vi "Set FTDI LatencyTimer.vi"() -> ()   [LabVIEW 2013]
uses:
  <vilib>/registry/registry.llb/Registry RtKey.ctl
  <vilib>/registry/registry.llb/Registry SAM.ctl
  <vilib>/registry/registry.llb/Read Registry Value Simple U32.vi
  <vilib>/registry/registry.llb/Read Registry Value Simple STR.vi
  <vilib>/registry/registry.llb/Write Registry Value Simple U32.vi
  <vilib>/regexp/Match Regular Expression.xnode
panel:
  out "New LatencyTimer List":u32[](array[numeric])
  out "Device Registry List":string[](array[string])
  out "# of Connected FTDI Devices":u32
  in  "LatencyTimer":i32=1
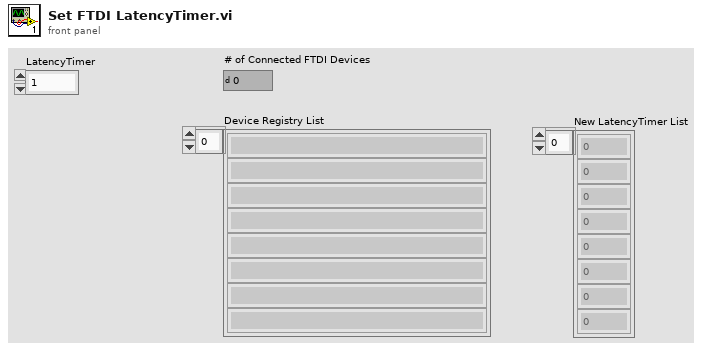
[diagram p1: front panel]
types:
  T1 = typedef "Registry SAM.ctl" = enum32{"KEY_QUERY_VALUE", "KEY_SET_VALUE", "KEY_CREATE_SUB_KEY", "KEY_ENUMERATE_SUB_KEYS", "KEY_NOTIFY", "KEY_CREATE_LINK", "KEY_READ", "KEY_WRITE", "KEY_ALL_ACCESS", "KEY_READ | KEY_WRITE"}
  T2 = typedef "Registry RtKey.ctl" = enum32{"HKEY_CLASSES_ROOT", "HKEY_CURRENT_USER", "HKEY_LOCAL_MACHINE", "HKEY_USERS", "HKEY_PERFORMANCE_DATA", "HKEY_CURRENT_CONFIG", "HKEY_DYN_DATA"}
  T3 = typedef "Registry refnum.ctl" = refnum<k1>
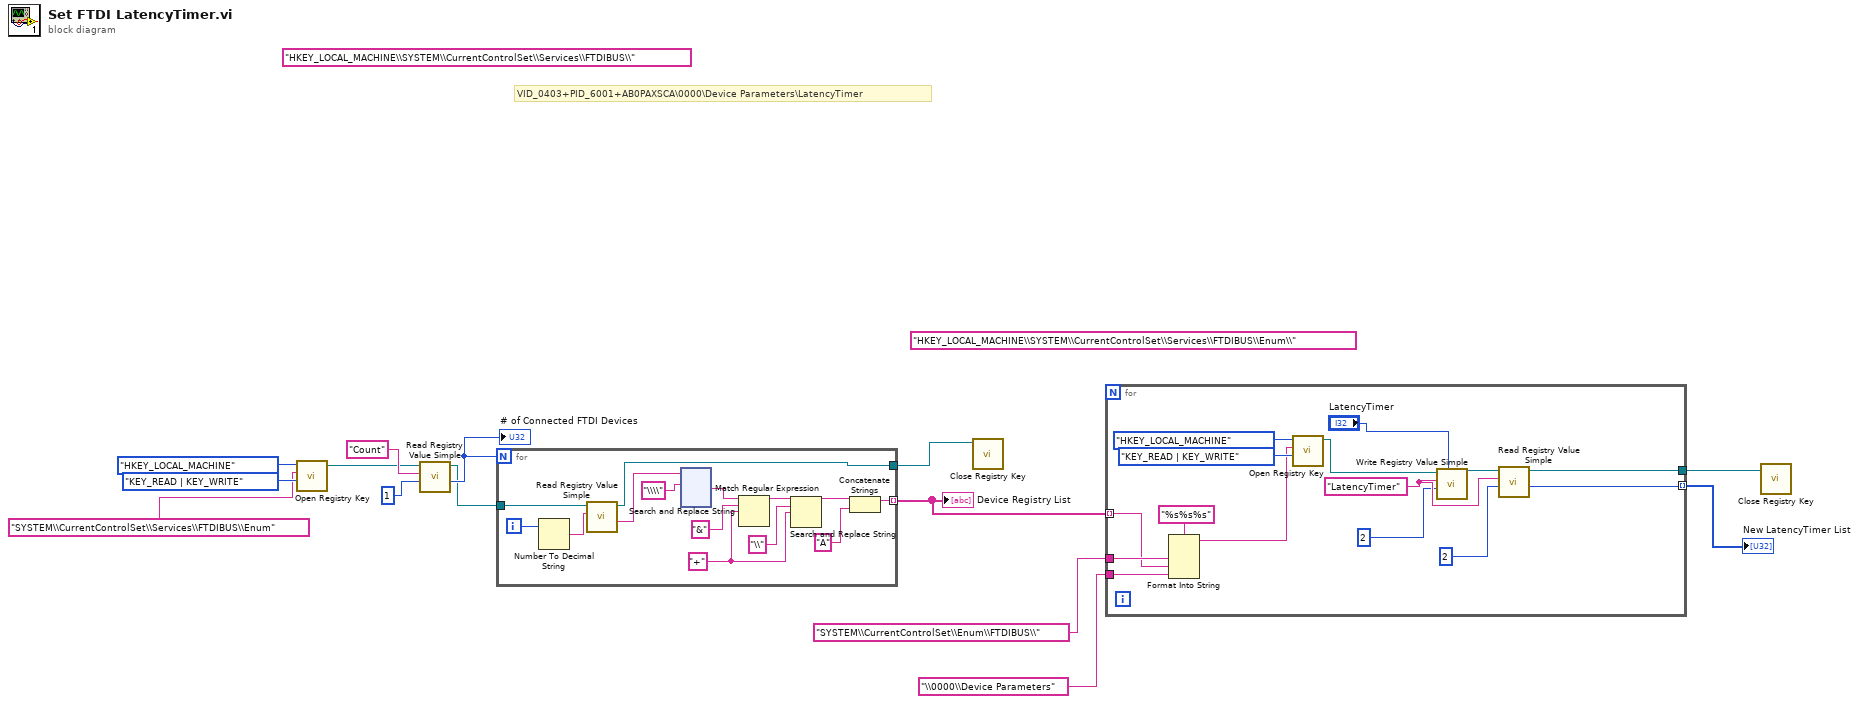
[diagram p0: block diagram]
diagram:
  (unwired) "HKEY_LOCAL_MACHINE\\SYSTEM\\CurrentControlSet\\Services\\FTDIBUS\\Enum\\" ("subkey")
  (unwired) "HKEY_LOCAL_MACHINE\\SYSTEM\\CurrentControlSet\\Services\\FTDIBUS\\" ("subkey")
  # "VID_0403+PID_6001+AB0PAXSCA\\0000\\Device Parameters\\LatencyTimer"
  n1 = call <vilib>:"Open Registry Key.vi"("security access mask (KEY_READ | KEY_WRITE)"=Registry_SAM."KEY_READ | KEY_WRITE", "subkey"="SYSTEM\\CurrentControlSet\\Services\\FTDIBUS\\Enum", "root key (HKEY_LOCAL_MACHINE)"=Registry_RtKey."HKEY_LOCAL_MACHINE") -> ("refnum out"=w10:T3)  [unwired: 7 in, 1 out]
  n2 = call-poly <vilib>:"Read Registry Value Simple.vi"("default data"=1, "value"="Count", "refnum"=w10) -> ("DWORD data"=w8:u32, "refnum out"=w7:T3)  [unwired: 3 in, 2 out]
  "# of Connected FTDI Devices" <- w8
  n3 = for {
    N: w8 -> [_]
    tunnel: w7 -> [w27]
    tunnel: [w15] -> w4 mode=indexing
    tunnel: [w18] -> w1
    i -> [w28]
    w20 = "+" ("search string")
    n4 = Number To Decimal String(number=w28) -> (decimal integer string=w26:string)  [unwired: 1 in]
    n5 = call-poly <vilib>:"Read Registry Value Simple.vi"("value"=w26, "refnum"=w27) -> ("String/Binary data"=w25:string, "refnum out"=w18:T3)  [unwired: 4 in, 2 out]
    n6 = xnode "Match Regular Expression"("input string"=w25, "regular expression"="\\\\") -> ("after match"=w24:string)  [unwired: 4 in, 4 out]
    n7 = Search and Replace String(input string=w24, search string="&" ("replace string (\"\")"), replace string=w20) -> (result string=w23:string)  [unwired: 5 in, 3 out]
    n8 = Search and Replace String(input string=w23, search string="\\", replace string=w20) -> (result string=w17:string)  [unwired: 5 in, 3 out]
    n9 = Concatenate Strings(w17, "A" ("string")) -> (w15:string)
  }
  "Device Registry List" <- w4
  n10 = call <vilib>:"Close Registry Key.vi"("refnum"=w1) -> ()  [unwired: 6 in, 1 out]
  n11 = for {
    tunnel: "SYSTEM\\CurrentControlSet\\Enum\\FTDIBUS\\" -> [w156]
    tunnel: "\\0000\\Device Parameters" -> [w155]
    tunnel: w4 -> [w151] mode=indexing
    tunnel: [w145] -> w3 mode=indexing
    tunnel: [w144] -> w2
    w147 = "LatencyTimer" ("value")
    n12 = Format Into String(format string="%s%s%s", w156, w151, w155) -> (resulting string=w152:string)  [unwired: 2 in, 1 out]
    n13 = call <vilib>:"Open Registry Key.vi"("security access mask (KEY_READ | KEY_WRITE)"=Registry_SAM."KEY_READ | KEY_WRITE", "subkey"=w152, "root key (HKEY_LOCAL_MACHINE)"=Registry_RtKey."HKEY_LOCAL_MACHINE") -> ("refnum out"=w149:T3)  [unwired: 7 in, 1 out]
    n14 = call-poly <vilib>:"Write Registry Value Simple.vi"("DWORD data"="LatencyTimer", "simple data type"=2, "value"=w147, "refnum"=w149) -> ("refnum out"=w148:T3)  [unwired: 4 in, 1 out]
    n15 = call-poly <vilib>:"Read Registry Value Simple.vi"("default data"=2, "value"=w147, "refnum"=w148) -> ("DWORD data"=w145:u32, "refnum out"=w144:T3)  [unwired: 3 in, 2 out]
  }
  "New LatencyTimer List" <- w3
  n16 = call <vilib>:"Close Registry Key.vi"("refnum"=w2) -> ()  [unwired: 6 in, 1 out]
